vi "write to RF synth bd - no WR.vi"(0 "Address Byte":u8, 1 "BD 2 Byte":u8, 2 "BD 1 Byte":u8) -> ()   [LabVIEW 2012]
uses:
  <vilib>/rvi/eio/common/nirviEmuTemplateMethod_errors.vi
  <vilib>/eio/EIONode/EIONode.xnode
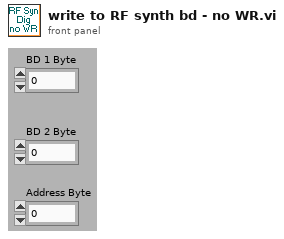
[diagram p1: front panel]
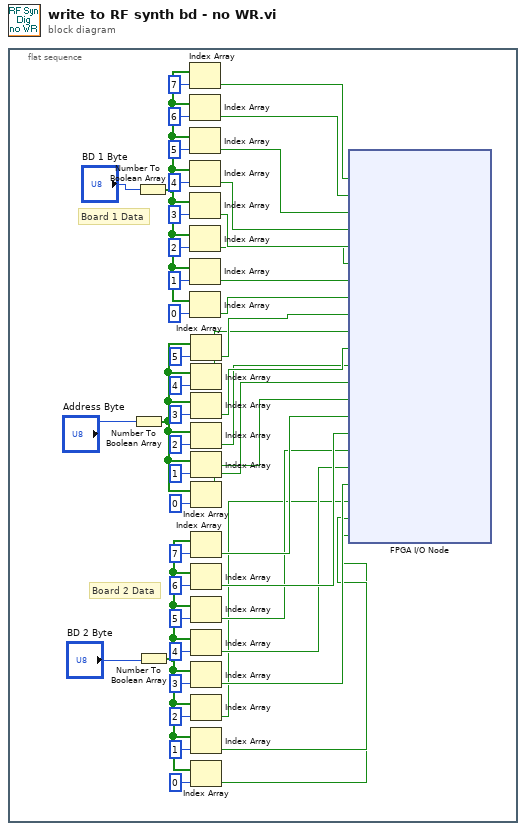
[diagram p0: block diagram]
diagram:
  n1 = flat-sequence {
    frame #0 {
      # "Board 1 Data"
      # "Board 2 Data"
      n2 = Number To Boolean Array(number="Address Byte") -> (Boolean array=w49:bool[])
      n3 = Number To Boolean Array(number="BD 1 Byte") -> (Boolean array=w50:bool[])
      n4 = Number To Boolean Array(number="BD 2 Byte") -> (Boolean array=w20:bool[])
      n5 = Index Array(array=w50, index=7) -> (element=w34:bool)
      n6 = Index Array(array=w50, index=6) -> (element=w33:bool)
      n7 = Index Array(array=w50, index=5) -> (element=w32:bool)
      n8 = Index Array(array=w50, index=4) -> (element=w31:bool)
      n9 = Index Array(array=w50, index=3) -> (element=w30:bool)
      n10 = Index Array(array=w50, index=2) -> (element=w29:bool)
      n11 = Index Array(array=w50, index=1) -> (element=w28:bool)
      n12 = Index Array(array=w50, index=0) -> (element=w27:bool)
      n13 = Index Array(array=w49, index=5) -> (element=w26:bool)
      n14 = Index Array(array=w49, index=4) -> (element=w25:bool)
      n15 = Index Array(array=w49, index=3) -> (element=w24:bool)
      n16 = Index Array(array=w49, index=2) -> (element=w23:bool)
      n17 = Index Array(array=w49, index=1) -> (element=w22:bool)
      n18 = Index Array(array=w49, index=0) -> (element=w21:bool)
      n19 = Index Array(array=w20, index=7) -> (element=w11:bool)
      n20 = Index Array(array=w20, index=6) -> (element=w10:bool)
      n21 = Index Array(array=w20, index=5) -> (element=w9:bool)
      n22 = Index Array(array=w20, index=4) -> (element=w8:bool)
      n23 = Index Array(array=w20, index=3) -> (element=w7:bool)
      n24 = Index Array(array=w20, index=2) -> (element=w6:bool)
      n25 = Index Array(array=w20, index=1) -> (element=w5:bool)
      n26 = Index Array(array=w20, index=0) -> (element=w4:bool)
      n27 = xnode "FPGA I/O Node"("Connector1/DIO0"=w34, "Connector1/DIO1"=w33, "Connector1/DIO2"=w32, "Connector1/DIO3"=w31, "Connector1/DIO4"=w30, "Connector1/DIO5"=w29, "Connector1/DIO6"=w28, "Connector1/DIO7"=w27, "Connector1/DIO8"=w26, "Connector1/DIO9"=w25, "Connector1/DIO10"=w24, "Connector1/DIO11"=w23, "Connector1/DIO12"=w22, "Connector1/DIO13"=w21, "Connector1/DIO20"=w11, "Connector1/DIO21"=w10, "Connector1/DIO22"=w9, "Connector1/DIO23"=w8, "Connector1/DIO24"=w7, "Connector1/DIO25"=w6, "Connector1/DIO26"=w5, "Connector1/DIO27"=w4) -> ()  [unwired: 22 in, 22 out]
    }
  }
